vi "Create Auto-Populating Folder.vi"(0 "project path":path, 5 "plug-in name":string, 11 "error in":errorcluster) -> (4 "measurement core reference":refnum<vi>, 6 "folder reference":refnum<vi>, 8 "project reference":refnum<vi>, 15 "error out":errorcluster)   [LabVIEW 2021, in "Multiple Converter.lvlib"]
uses:
  Multiple Converter.lvlib
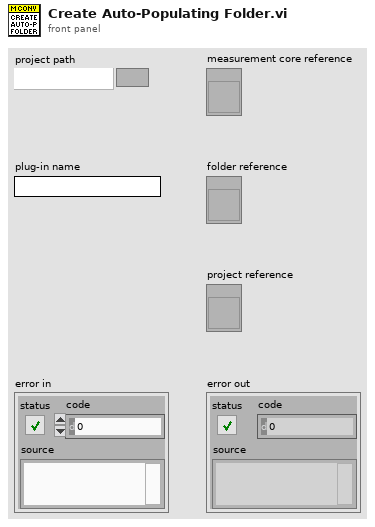
[diagram p1: front panel]
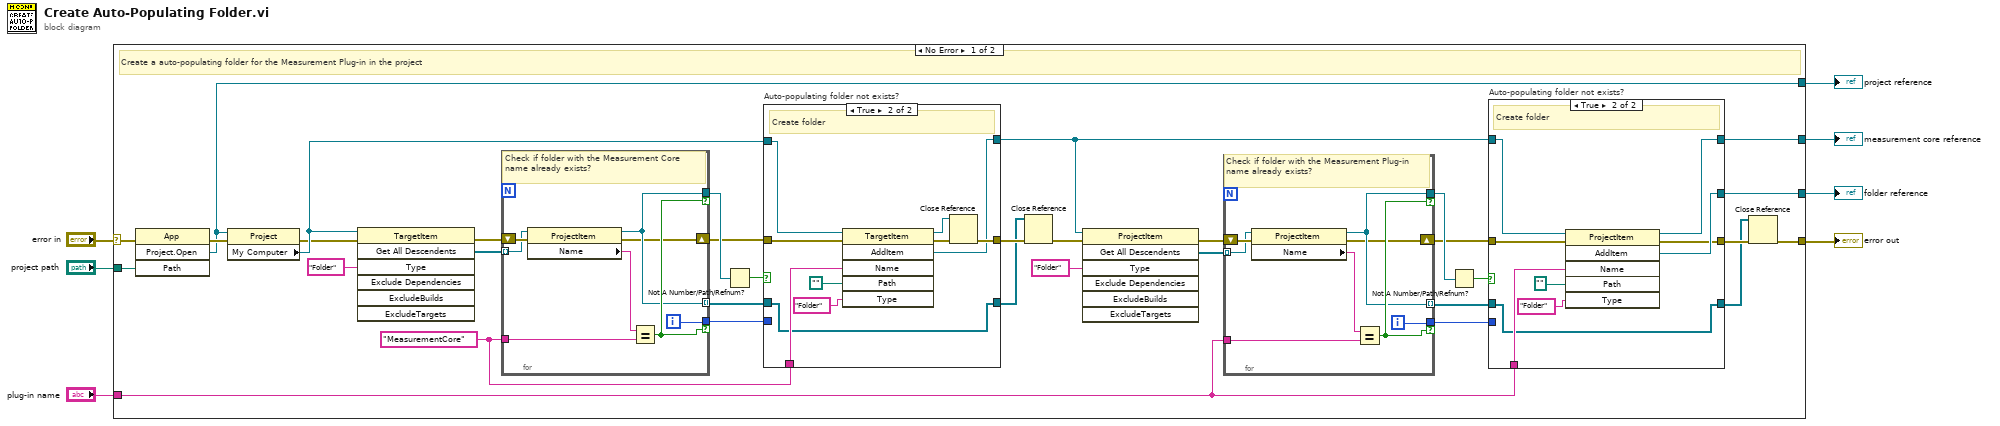
[diagram p0: block diagram]
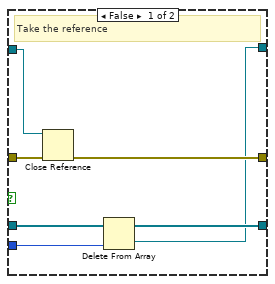
[diagram p2: hidden frame]
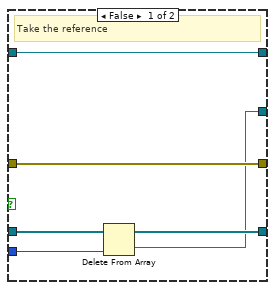
[diagram p3: hidden frame]
diagram:
  n1 = case shown="No Error" "error in" {
    selector: "error in" -> [w37 w89]
    tunnel: [w11 w89] -> w7
    tunnel: "project path" -> [w31 _]
    tunnel: "plug-in name" -> [w16 _]
    tunnel: [w14 _] -> w4
    tunnel: [w13 _] -> w3
    tunnel: [w12 _] -> w2
    frame No Error {
      w10 = "MeasurementCore"
      # "Create a auto-populating folder for the Measurement Plug-in in the project"
      n2 = invoke class="App" method="Project.Open"(error in=w37, "Path"=w31) -> (error out=w33:errorcluster, "Project:Open"=w12:refnum<vi>)  [unwired: 2 in, 2 out]
      n3 = property class="Project"(reference=w12, error in=w33) -> (error out=w34:errorcluster, "My Computer"=w39:refnum<vi>)  [unwired: 1 out]
      n4 = invoke class="TargetItem" method="Get All Descendents"(reference=w39, error in=w34, "Type"="Folder") -> (error out=w36:errorcluster, "All Descendents"=w32:refnum<vi>[])  [unwired: 4 in, 5 out]
      n5 = for {
        tunnel: w32 -> [w47] mode=indexing
        tunnel: [w42] -> w28 if=w43
        tunnel: w10 -> [w45]
        tunnel: [w44] -> w30 if=w43
        tunnel: [w42] -> w29 mode=indexing
        shift-right: [w41] -> w9
        shift-left: w36 -> [w48]
        i -> [w44]
        # "Check if folder with the Measurement Core name already exists?"
        n6 = property class="ProjectItem"(reference=w47, error in=w48) -> (reference out=w42:refnum<vi>, error out=w41:errorcluster, "Name"=w46:string)
        n7 = Equal?(x=w46, y=w45) -> (x = y?=w43:bool)
      }
      n8 = Not A Number/Path/Refnum?(number/path/refnum=w28) -> (NaN/Path/Refnum?=w38:bool)
      n9 = case "Auto-populating folder not exists?" shown="True" w38 {
        tunnel: w39 -> [w53 w65]
        tunnel: w9 -> [w55 w61]
        tunnel: [w54 w60] -> w40
        tunnel: w10 -> [_ w58]
        tunnel: [w49 w57] -> w15
        tunnel: w30 -> [w51 _]
        tunnel: w29 -> [w52 w56]
        tunnel: [w50 w56] -> w27
        frame False {
          # "Take the reference"
          n10 = Close Reference(reference=w53, error in (no error)=w55) -> (error out=w54:errorcluster)
          n11 = Delete From Array(array=w52, index=w51) -> (deleted portion=w49:refnum<vi>, array with subset deleted=w50:refnum<vi>[])  [unwired: 1 in]
        }
        frame True {
          # "Create folder"
          n12 = invoke class="TargetItem" method="AddItem"(reference=w65, error in=w61, "Name"=w58, "Path"=path "", "Type"="Folder") -> (reference out=w62:refnum<vi>, error out=w63:errorcluster, "AddItem"=w57:refnum<vi>)  [unwired: 1 in, 3 out]
          n13 = Close Reference(reference=w62, error in (no error)=w63) -> (error out=w60:errorcluster)
        }
      }
      n14 = Close Reference(reference=w27, error in (no error)=w40) -> (error out=w18:errorcluster)
      n15 = invoke class="ProjectItem" method="Get All Descendents"(reference=w15, error in=w18, "Type"="Folder") -> (error out=w24:errorcluster, "All Descendents"=w23:refnum<vi>[])  [unwired: 4 in, 5 out]
      n16 = for {
        tunnel: w23 -> [w72] mode=indexing
        tunnel: [w67] -> w20 if=w68
        tunnel: w16 -> [w70]
        tunnel: [w69] -> w22 if=w68
        tunnel: [w67] -> w21 mode=indexing
        shift-right: [w66] -> w8
        shift-left: w24 -> [w73]
        i -> [w69]
        # "Check if folder with the Measurement Plug-in name already exists?"
        n17 = property class="ProjectItem"(reference=w72, error in=w73) -> (reference out=w67:refnum<vi>, error out=w66:errorcluster, "Name"=w71:string)
        n18 = Equal?(x=w71, y=w70) -> (x = y?=w68:bool)
      }
      n19 = Not A Number/Path/Refnum?(number/path/refnum=w20) -> (NaN/Path/Refnum?=w25:bool)
      n20 = case "Auto-populating folder not exists?" shown="True" w25 {
        tunnel: w8 -> [w79 w87]
        tunnel: [w79 w81] -> w26
        tunnel: w16 -> [_ w85]
        tunnel: [w75 w84] -> w14
        tunnel: w22 -> [w77 _]
        tunnel: w21 -> [w78 w83]
        tunnel: [w76 w83] -> w19
        tunnel: w15 -> [w74 w82]
        tunnel: [w74 w80] -> w13
        frame False {
          # "Take the reference"
          n21 = Delete From Array(array=w78, index=w77) -> (deleted portion=w75:refnum<vi>, array with subset deleted=w76:refnum<vi>[])  [unwired: 1 in]
        }
        frame True {
          # "Create folder"
          n22 = invoke class="ProjectItem" method="AddItem"(reference=w82, error in=w87, "Name"=w85, "Path"=path "", "Type"="Folder") -> (reference out=w80:refnum<vi>, error out=w81:errorcluster, "AddItem"=w84:refnum<vi>)  [unwired: 1 in, 3 out]
        }
      }
      n23 = Close Reference(reference=w19, error in (no error)=w26) -> (error out=w11:errorcluster)
    }
    frame Error {
    }
  }
  "error out" <- w7
  "folder reference" <- w4
  "measurement core reference" <- w3
  "project reference" <- w2
